vi "Receive Message.vi"(6 "priority":i32, 10 "MailboxClient in":refnum<class "MailboxClient.lvclass">, 11 "Message in":refnum<class "Message.lvclass">) -> (0 "error out":errorcluster, 2 "Actor out":refnum<class "Actor.lvclass">)   [LabVIEW 2020, in "MailboxClient.lvlib" / "MailboxClient.lvclass"]
doc: "This VI should be overriden ONLY if you are creating a proxy actor for remote transmission. If you are, override this VI to transmit the received message to a new destination, maintaining the given priority."
uses:
  MailboxClient.lvclass
  <vilib>/ActorFramework/Actor/Actor.lvclass
  MailboxManager/_Msg-Filter/_Msg-Filter.lvclass
  <vilib>/ActorFramework/Message/Message.lvclass
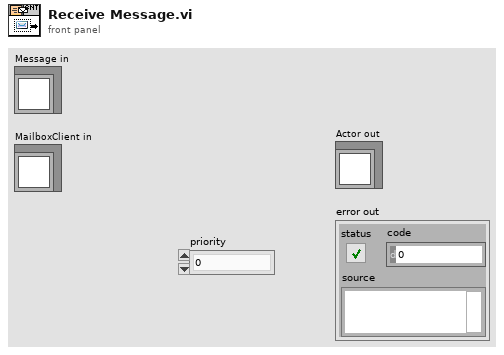
[diagram p1: front panel]
types:
  T1 = map{refnum<class "Message.lvclass">, refnum<class "_Msg-Filter.lvclass">}
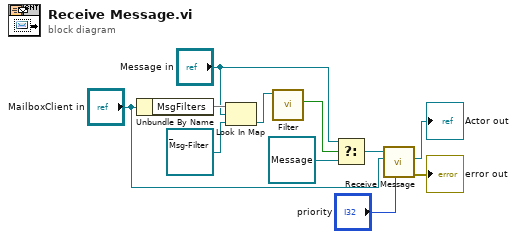
[diagram p0: block diagram]
diagram:
  n1 = Unbundle By Name("MailboxClient in") -> ("MsgFilters"=w7:T1)
  n2 = Look In Map(map=w7, key="Message in", default value=refnum<class "_Msg-Filter.lvclass"> refnum ("MailboxClient.lvlib:_Msg-Filter.lvclass")) -> (value=w6:refnum<class "_Msg-Filter.lvclass">)  [unwired: 1 out]
  n3 = call-dynamic "Filter.vi"("_Msg-Filter in"=w6) -> ("Found?"=w4:bool)  [unwired: 9 in, 1 out]
  n4 = Select(t="Message in", s=w4, f=refnum<class "Message.lvclass"> refnum ("Message")) -> (s? t:f=w1:refnum<class "Message.lvclass">)
  n5 = call-parent "Receive Message.vi"("priority"="priority", "Actor in"="MailboxClient in", "Message in"=w1) -> ("error out"=→"error out":errorcluster, "Actor out"=→"Actor out":refnum<class "Actor.lvclass">)  [unwired: 7 in]
